vi "DecodeFlags.vi"(8 "error in":errorcluster, 10 "Array":u8[](array[numeric]) format="%02x") -> (0 "error IO":errorcluster, 2 "array w/ subset deleted":u8[](array[numeric]), 3 "Flags":bool[](array[boolean]))   [LabVIEW 2017]
uses:
  Varint Decoder uint32.vi
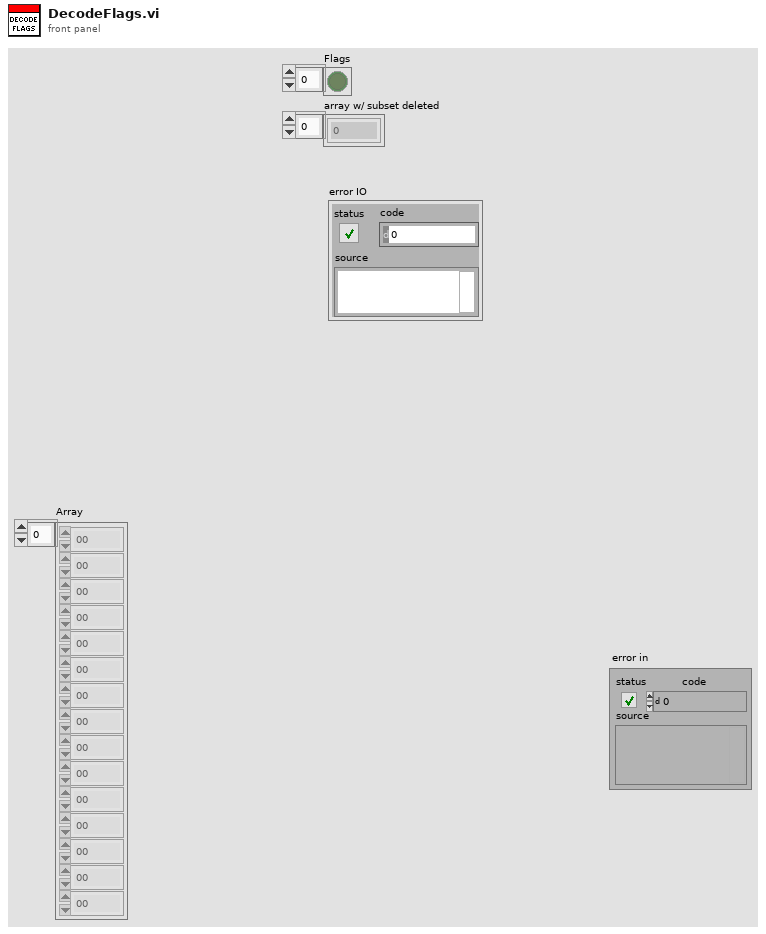
[diagram p1: front panel]
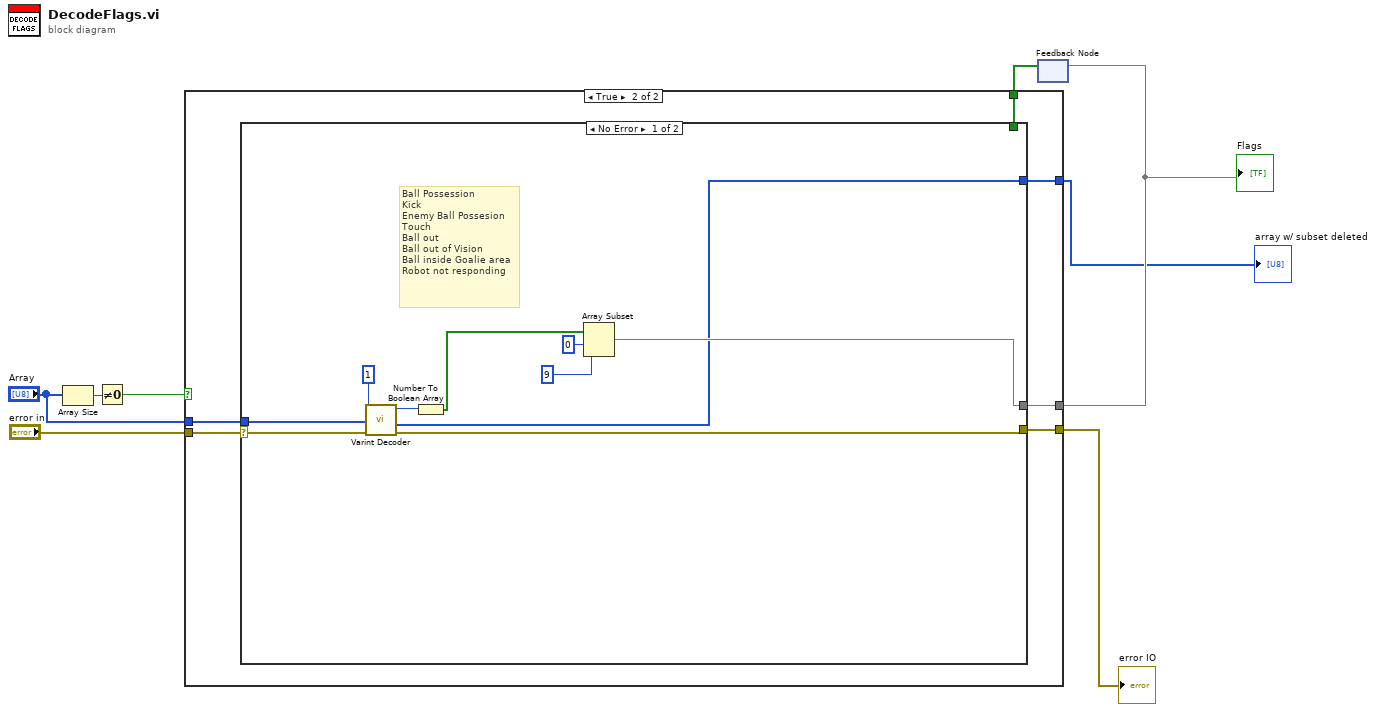
[diagram p0: block diagram]
diagram:
  n1 = Array Size(array="Array") -> (size(s)=w8:i32)
  n2 = Not Equal To 0?(x=w8) -> (x != 0?=w7:bool)
  n3 = feedback #1() -> (w2:bool[])  [unwired: 1 in]
  n4 = case shown="True" w7 {
    tunnel: "error in" -> [w11 w17]
    tunnel: "Array" -> [w10 w16]
    tunnel: [w11 w15] -> w4
    tunnel: [w10 w12] -> w1
    tunnel: [w9 w14] -> w3
    tunnel: w2 -> [w9 w13]
    frame False {
    }
    frame True {
      n5 = case shown="No Error" w17 {
        selector: w17 -> [w25 w30]
        tunnel: w16 -> [w27 w29]
        tunnel: [w24 w30] -> w15
        tunnel: [w18 w29] -> w12
        tunnel: [w19 w28] -> w14
        tunnel: w13 -> [_ w28]
        frame No Error {
          # "Ball Possession\nKick\nEnemy Ball Possesion\nTouch\nBall out\nBall out of Vision\nBall inside Goalie area\nRobot not responding"
          n6 = call-poly "Varint Decoder.vi"("error in (no error)"=w25, "Array"=w27, "Key"=1) -> ("error out"=w24:errorcluster, "array w/ subset deleted"=w18:u8[], "Varint"=w23:u32)  [unwired: 5 in, 1 out]
          n7 = Number To Boolean Array(number=w23) -> (Boolean array=w22:bool[])
          n8 = Array Subset(array=w22, index=0, length=9) -> (w19:bool[])
        }
        frame Error {
        }
      }
    }
  }
  "error IO" <- w4
  "Flags" <- w3
  "array w/ subset deleted" <- w1
  n9 = feedback-in #1(w3) -> ()
